vi "Prediction Interval (Linear).vi"(0 "Y":dbl[](array[numeric]), 1 "confidence level":dbl=0.95 format="%.2f", 5 "X":dbl[](array[numeric]), 7 "Weight":dbl[](array[numeric]), 9 "slope":dbl, 11 "intercept":dbl) -> (4 "Upper Bound":dbl[](array[numeric]), 6 "Lower Bound":dbl[](array[numeric]), 15 "error":i32)   [LabVIEW 2020, in "NI_AALPro.lvlib"]
doc: "Calculates statistical intervals of the best linear fit for a data set (<B>X</B>, <B>Y</B>). You must manually select the polymorphic instance to use."
uses:
  NI_AALPro.lvlib
  <resource>/lvanlys.dll
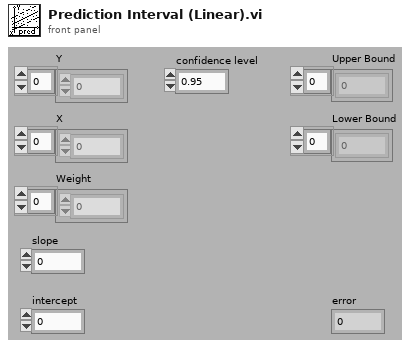
[diagram p1: front panel]
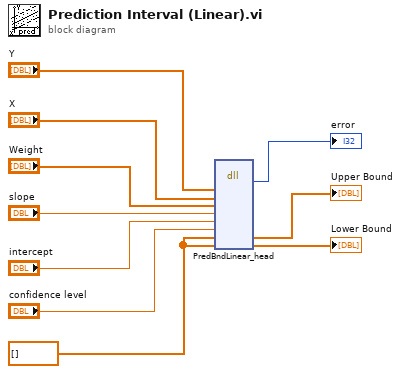
[diagram p0: block diagram]
diagram:
  w2 = dbl[] [] ("Best Linear Fit")
  n1 = dll-call lib="C:/Program Files (x86)/National Instruments/LabVIEW 2020/resource/lvanlys.*" fn="PredBndLinear_head"("y"="Y", "x"="X", "weight"="Weight", "slope"="slope", "intercept"="intercept", "confidentLevel"="confidence level", "upper"=w2, "lower"=w2) -> (→"error":i32, "upper"=→"Upper Bound":dbl[], "lower"=→"Lower Bound":dbl[])  [unwired: 9 in, 2 out]
